vi "Trial data array-Build.vi"(5 "Total number of points acquired":i32, 7 "Target number of points":u32, 8 "error in":errorcluster, 9 "Buffer (in)":dbl[](array[numeric]), 10 "Logging queue element":T1={"Imaging Protocol"=enum."Live Imaging", "Number of Trials"=0, "Frame Size"=512, "# Averaged frames"=0, "Dwell time (us)"=0.0, "Index of Z-plane"=0, "Timelapse?"=FALSE, "Logging process is active"=FALSE, "Speed logging enabled"=FALSE, "tdms file ref"=refnum, "path"=path "", "Trial Number"=0, "Expected # points acquired"=FALSE, "Manually stopped"=FALSE, "Ch0 data"=[], "Ch1 data"=[], "Ref Data"=[], "Last trial"=FALSE, "Ref Dwell time (us)"=0.0, "# Ref Averaged frames"=0, "Ref X Length"=0, "Ref Y Length"=0, "Points acquired"={"Ch0 last trial"=0, "Ch1 last trial"=0, "All trials"=0}} {"Ref Dwell time (us)" format="%#.6g"; "Frame Size" items=["100X100"=100, "128X128"=128, "200X200"=200, "256X256"=256, "512X512"=512, "1024x1024"=1024, "2048x2048"=2048]; "Dwell time (us)" format="%#.6g"}, 11 "Chunk of data (in)":dbl[](array[numeric])) -> (1 "Buffer (out) / Full frame data when in Z-stack mode":dbl[](array[numeric]))   [LabVIEW 2017]
uses:
  Typedefs/Logging queue element.ctl
  Typedefs/Imaging Protocols enum.ctl
  Typedefs/Frame Size.ctl
  Typedefs/Acquired points count.ctl
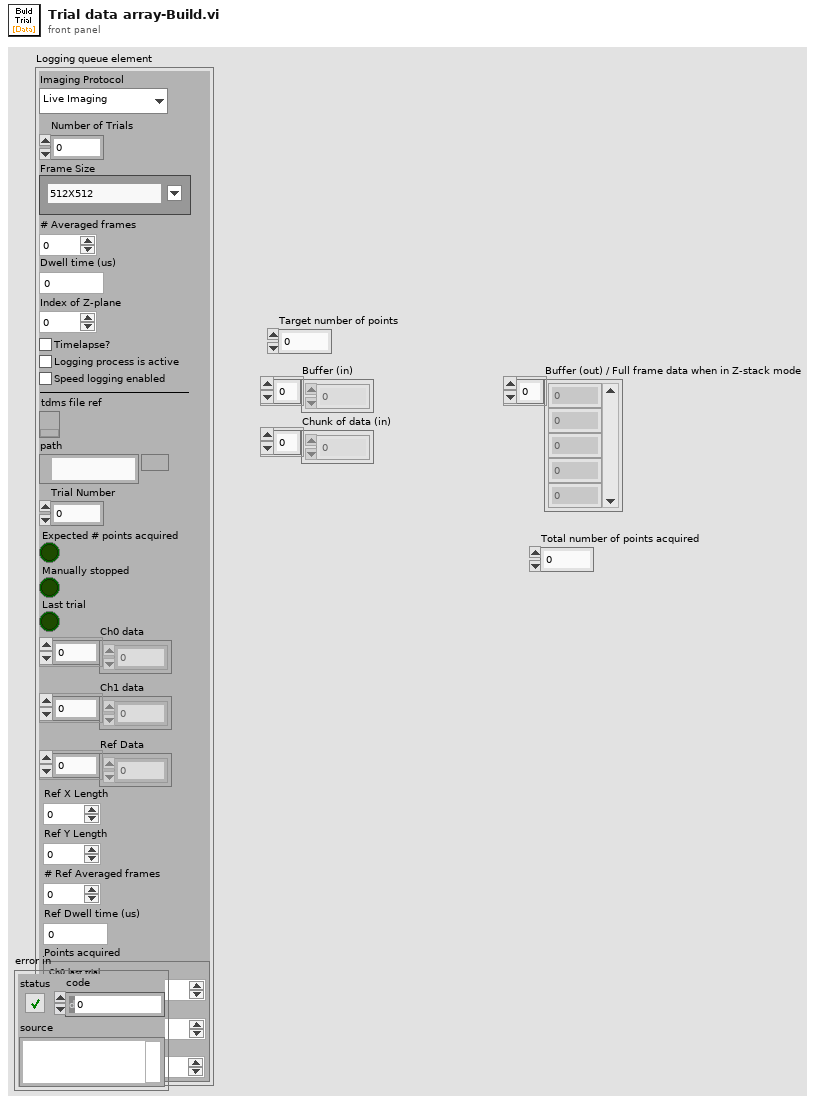
[diagram p1: front panel]
types:
  T1 = typedef "Logging queue element.ctl" = cluster{"Imaging Protocol":T2, "Number of Trials":u16, "Frame Size":T3, "# Averaged frames":u16, "Dwell time (us)":dbl, "Index of Z-plane":i32, "Timelapse?":bool, "Logging process is active":bool, "Speed logging enabled":bool, "tdms file ref":refnum<k34>, "path":path, "Trial Number":i32, "Expected # points acquired":bool, "Manually stopped":bool, "Ch0 data":u32[], "Ch1 data":u32[], "Ref Data":u32[], "Last trial":bool, "Ref Dwell time (us)":dbl, "# Ref Averaged frames":u16, "Ref X Length":u16, "Ref Y Length":u16, "Points acquired":T4}
  T2 = typedef "Imaging Protocols enum.ctl" = enum16{"AOL Z-Stack", "Motor Z Stack", "Functional Acquisition", "Single Plane Acquisition", "Volume Acquisition", "Live Imaging", "Live Plane Imaging", "Live Volume Imaging"}
  T3 = typedef "Frame Size.ctl" = u16
  T4 = typedef "Acquired points count.ctl" = cluster{"Ch0 last trial":u64, "Ch1 last trial":u64, "All trials":u64}
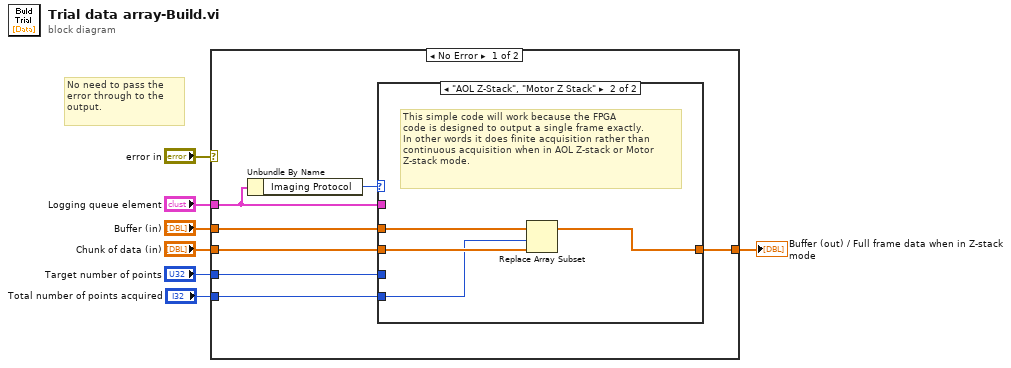
[diagram p0: block diagram]
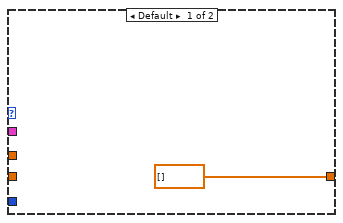
[diagram p2: hidden frame]
diagram:
  # "No need to pass the error through to the output."
  n1 = case shown="No Error" "error in" {
    tunnel: "Logging queue element" -> [w8 _]
    tunnel: [w13 w20] -> w6
    tunnel: "Buffer (in)" -> [w12 _]
    tunnel: "Chunk of data (in)" -> [w11 w20]
    tunnel: "Target number of points" -> [w10 _]
    tunnel: "Total number of points acquired" -> [w9 _]
    frame No Error {
      n2 = Unbundle By Name(w8) -> ("Imaging Protocol"=w14:T2)
      n3 = case shown="\"AOL Z-Stack\", \"Motor Z Stack\"" w14 {
        tunnel: w12 -> [_ w18]
        tunnel: [dbl[] [] ("Buffer (in)") w19] -> w13
        tunnel: w11 -> [_ w17]
        tunnel: w10 -> [_ _]
        tunnel: w9 -> [_ w16]
        tunnel: w8 -> [_ _]
        frame Default {
        }
        frame "AOL Z-Stack", "Motor Z Stack" {
          # "This simple code will work because the FPGA \ncode is designed to output a single frame exactly.\nIn other words it does finite acquisition rather than continuous acquisition when in AOL Z-stack or Motor Z-stack mode."
          n4 = Replace Array Subset "Replace Array Subset"(array=w18, new element=w17, index=w16) -> (w19:dbl[])
        }
      }
    }
    frame Error {
    }
  }
  "Buffer (out) / Full frame data when in Z-stack mode" <- w6
